vi "POP_Breakout Controls to Register.vi"(11 "Popup":refnum<vi>) -> (1 "Color & Ring":refnum<vi>[](array[refnum]), 3 "Unknown":refnum<vi>, 4 "Clusters OK":refnum<vi>[](array[refnum]), 6 "Clusters Cancel":refnum<vi>[](array[refnum]))   [LabVIEW 2016]
uses:
  Ctrls/POP_Data Type.ctl
panel:
  in  "error in (no error)":errorcluster
  out "error out":errorcluster
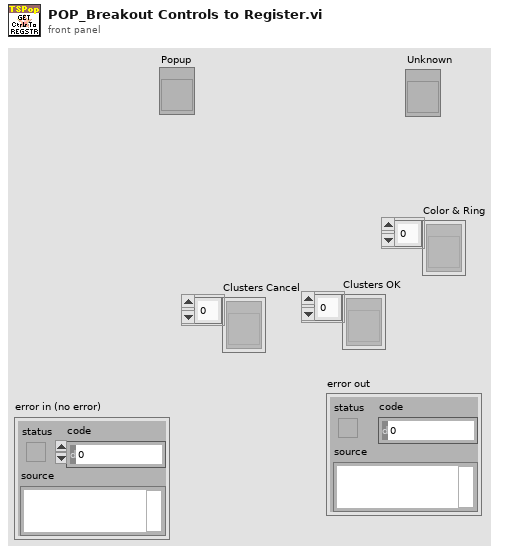
[diagram p1: front panel]
types:
  T1 = typedef "POP_Data Type.ctl" = enum16{"NO POPUP", "Unkown", "String", "Integer", "Float", "Color", "Boolean", "Ring", "Captioned String", "Captioned Integer", "Button Color", "2 Int Cluster", "4 Int Cluster", "6-Dbl Cluster", "Path", "Combox", "Time", "ShotCut String"}
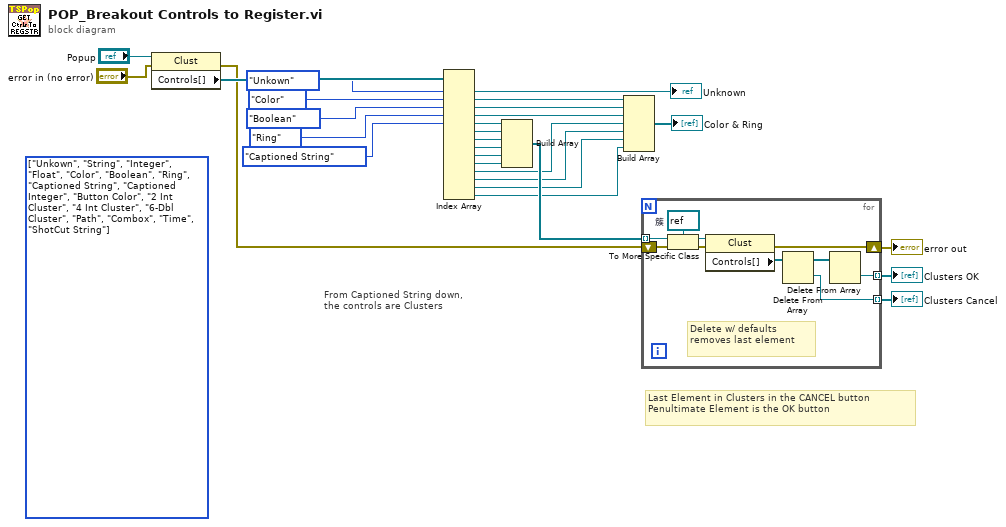
[diagram p0: block diagram]
diagram:
  (unwired) T1[] [enum."Unkown", enum."String", enum."Integer", enum."Float", enum."Color", enum."Boolean", enum."Ring", enum."Captioned String", enum."Captioned Integer", enum."Button Color", enum."2 Int Cluster", enum."4 Int Cluster", enum."6-Dbl Cluster", enum."Path", enum."Combox", enum."Time", enum."ShotCut String"] items=["NO POPUP", "Unkown", "String", "Integer", "Float", "Color", "Boolean", "Ring", "Captioned String", "Captioned Integer", "Button Color", "2 Int Cluster", "4 Int Cluster", "6-Dbl Cluster", "Path", "Combox", "Time", "ShotCut String"]
  # "Last Element in Clusters in the CANCEL button\nPenultimate Element is the OK button"
  # "From Captioned String down,\nthe controls are Clusters"
  n1 = property class="Clust"(reference="Popup", error in="error in (no error)") -> (error out=w8:errorcluster, "Controls[]"=w27:refnum<vi>[])  [unwired: 1 out]
  n2 = Index Array(array=w27, index #1=POP_Data_Type."Unkown" ("Prop Type"), index #2=POP_Data_Type."Color" ("Prop Type"), index #3=POP_Data_Type."Boolean" ("Prop Type"), index #4=POP_Data_Type."Ring" ("Prop Type"), index #5=POP_Data_Type."Captioned String" ("Prop Type")) -> (element #1=→"Unknown":refnum<vi>, element #2=w10:refnum<vi>, element #3=w25:refnum<vi>, element #4=w24:refnum<vi>, element #5=w22:refnum<vi>, element #6=w21:refnum<vi>, element #7=w20:refnum<vi>, element #8=w19:refnum<vi>, element #9=w18:refnum<vi>, element #10=w5:refnum<vi>, element #11=w4:refnum<vi>, element #12=w3:refnum<vi>, element #13=w2:refnum<vi>, element #14=w1:refnum<vi>)  [unwired: 9 in]
  n3 = Build Array(w22, w21, w20, w19, w18, w5) -> (w17:refnum<vi>[])
  n4 = Build Array(w10, w25, w24, w4, w3, w2, w1) -> (→"Color & Ring":refnum<vi>[])
  n5 = for {
    tunnel: w17 -> [w38] mode=indexing
    tunnel: [w33] -> w15 mode=indexing
    tunnel: [w31] -> w16 mode=indexing
    shift-right: [w30] -> w7
    shift-left: w8 -> [w29]
    w37 = refnum<vi> refnum  # 簇
    # "Delete w/ defaults\nremoves last element"
    n6 = To More Specific Class(target class=w37, reference=w38, error in=w29) -> (specific class reference=w36:refnum<vi>, error out=w35:errorcluster)
    n7 = property class="Clust"(reference=w36, error in=w35) -> (error out=w30:errorcluster, "Controls[]"=w34:refnum<vi>[])  [unwired: 1 out]
    n8 = Delete From Array(array=w34) -> (deleted portion=w33:refnum<vi>, array with subset deleted=w32:refnum<vi>[])  [unwired: 2 in]
    n9 = Delete From Array(array=w32) -> (deleted portion=w31:refnum<vi>)  [unwired: 2 in, 1 out]
  }
  "Clusters OK" <- w16
  "Clusters Cancel" <- w15
  "error out" <- w7
